vi "Dist Build App from LLB (proxy).vi"(4 "include run-time DLL":bool, 5 "active x server":string, 6 "mac mem size (k)":u32, 7 "lvrt res flags":i32, 8 "error in":errorcluster, 11 "paths":T1) -> (0 "error out":errorcluster)   [LabVIEW 2009]
doc: "\"Call By Reference\" proxy for .\\project\\prodisttol.llb\\Dist Build App from LLB.vi"
panel:
  in  "LV6.1 VI Refnum (for type)":refnum<vi>
  in  "LV7 VI Refnum (for type)":refnum<vi>
  in  "VI Refnum (for type)":refnum<vi>
  # "Dist Build App from LLB (proxy).vi\n\n\"Call By Reference\" proxy for .\\project\\prodisttol.llb\\Dist Build App from LLB.vi\n\nPlease visit http://www.OpenG.org to learn about the\nOpen Source LabVIEW software movement.\n\nNOTICE -- YOU MUST LEAVE THIS NOTICE IN PLACE.  PER THE TERMS OF THE LICENSE BELOW, YOU MAY SUBLICENSE THIS SOFTWARE \nIN ANY WAY THAT DOES NOT CONFLICT WITH THIS LICENSE.\n\n### BSD License (http://www.opensource.org/licenses/bsd-license.php) Begin ###\n \nCopyright (c) 2002, Jim Kring <jim@jimkring.com>\n\nAll rights reserved.\n\nRedistribution and use in source and binary forms, with or without modification, are permitted provided that the following conditions are met:\n\n    * Redistributions of source code must retain the above copyright notice, this list of conditions and the following disclaimer.\n    * Redistributions in binary form must reproduce the above copyright notice, this list of conditions and the following disclaimer in the \n       documentation and/or other materials provided with the distribution.\n    * Neither the name of SciWare, James Kring, Inc., nor the names of its contributors may be used to endorse or promote products derived \n       from this software without specific prior written permission.\n\nTHIS SOFTWARE IS PROVIDED BY THE COPYRIGHT HOLDERS AND CONTRIBUTORS \"AS IS\" AND ANY EXPRESS OR IMPLIED WARRANTIES, \nINCLUDING, BUT NOT LIMITED TO, THE IMPLIED WARRANTIES OF MERCHANTABILITY AND FITNESS FOR A PARTICULAR PURPOSE ARE \nDISCLAIMED. IN NO EVENT SHALL THE COPYRIGHT OWNER OR CONTRIBUTORS BE LIABLE FOR ANY DIRECT, INDIRECT, INCIDENTAL,\n SPECIAL, EXEMPLARY, OR CONSEQUENTIAL DAMAGES (INCLUDING, BUT NOT LIMITED TO, PROCUREMENT OF SUBSTITUTE GOODS OR \nSERVICES; LOSS OF USE, DATA, OR PROFITS; OR BUSINESS INTERRUPTION) HOWEVER CAUSED AND ON ANY THEORY OF LIABILITY, \nWHETHER IN CONTRACT, STRICT LIABILITY, OR TORT (INCLUDING NEGLIGENCE OR OTHERWISE) ARISING IN ANY WAY OUT OF THE USE \nOF THIS SOFTWARE, EVEN IF ADVISED OF THE POSSIBILITY OF SUCH DAMAGE.\n\n### BSD License End ###"
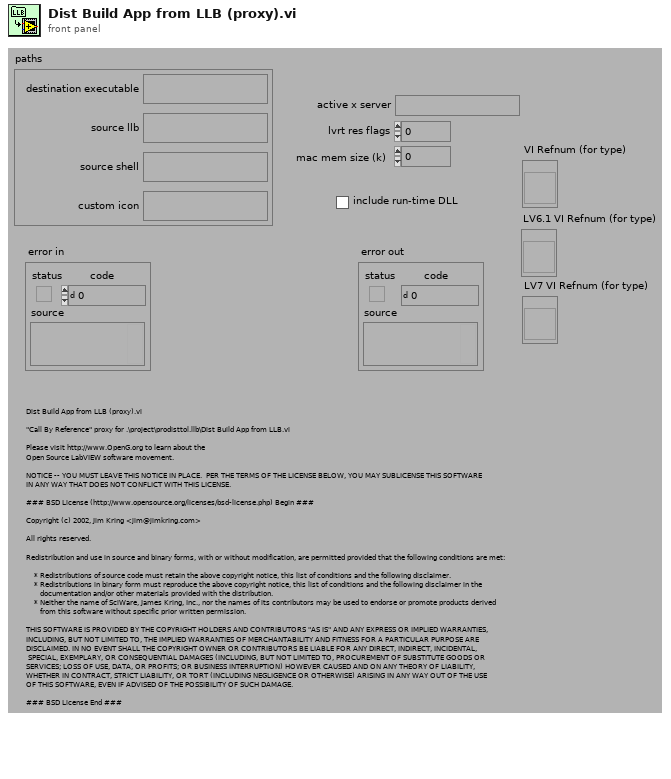
[diagram p1: front panel]
types:
  T1 = cluster{"destination executable":path, "source llb":path, "source shell":path, "custom icon":path}
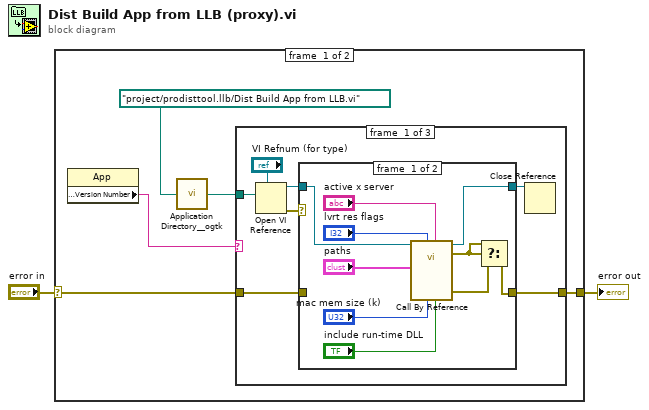
[diagram p0: block diagram]
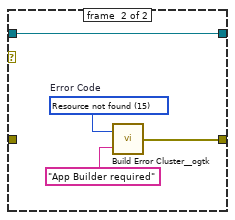
[diagram p2: hidden frame]
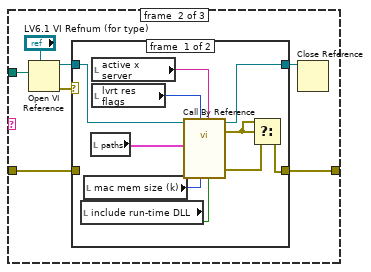
[diagram p3: hidden frame]
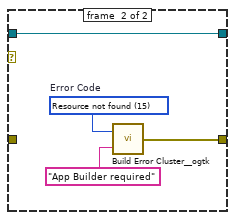
[diagram p4: hidden frame]
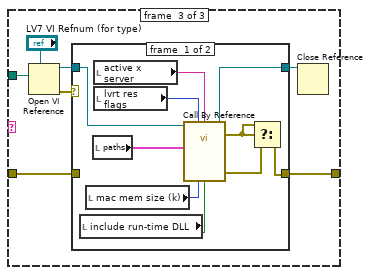
[diagram p5: hidden frame]
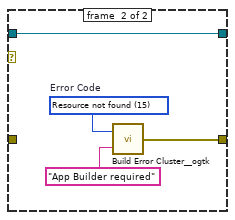
[diagram p6: hidden frame]
diagram:
  n1 = case shown="No Error" "error in" {
    selector: "error in" -> [w7 w71]
    tunnel: [w6 w71] -> w1
    frame #0 {
      n2 = property class="App"() -> ("Application:Version Number"=w5:string)  [unwired: 2 in, 2 out]
      n3 = call <userlib>:"Application Directory__ogtk.vi"("Relative path (.)"=path "project/prodisttool.llb/Dist Build App from LLB.vi") -> ("Application Directory (+ Relative)"=w4:path)
      n4 = case shown="\"6.0\", \"6.0.1\", \"6.0.2\"" w5 {
        tunnel: w4 -> [w14 w35 w56]
        tunnel: w7 -> [w12 w33 w54]
        tunnel: [w11 w32 w53] -> w6
        frame #0 {
          n5 = Open VI Reference(type specifier VI Refnum (for type only)="VI Refnum (for type)", vi path=w14) -> (vi reference=w10:refnum<vi>, error out=w13:errorcluster)  [unwired: 4 in]
          n6 = case shown="No Error" w13 {
            tunnel: w12 -> [_ _]
            tunnel: [w15 w27] -> w11
            tunnel: w10 -> [w24 w26]
            tunnel: [w18 w26] -> w8
            frame #0 {
              n7 = call-by-ref "?"(reference=w24, "include run-time DLL"="include run-time DLL", "active x server"="active x server", "mac mem size (k)"="mac mem size (k)", "lvrt res flags"="lvrt res flags", "paths"="paths") -> (reference out=w18:refnum<vi>, error out=w17:errorcluster, "error out"=w16:errorcluster)  [unwired: 7 in]
              n8 = Select(t=w17, s=w17, f=w16) -> (s? t:f=w15:errorcluster)
            }
            frame #1 {
              w25 = u16 15 items=["No error", "Argument error", "Memory is full", "Out of zone", "End of file", "File already open", "Generic file I/O error", "File not found", "File permission error", "Disk is full", "Duplicate path", "Too many files open", "System feature not enabled", "Resource file not found", "Cannot add resource", "Resource not found", "Image not found", "Image memory error", "Pen does not exist", "Config type invalid", "Config token not found", "Config parse error", "Config memory error", "Bad external code format", "Bad external code offset", "External code not present", "Null window", "Destroy window error", "Null menu", "Print aborted", "Bad print record", "Print driver error", "Windows error during printing", "Memory error during printing", "Print dialog error", "Generic print error", "Invalid device refnum", "Device not found", "Device parameter error", "Device unit error", "Cannot open device", "Device call aborted", "Generic error", "Cancelled by user", "Object ID too low", "Object ID too high", "Object not in heap", "Unknown heap", "Unknown object (invalid DefProc)", "Unknown object (DefProc not in table)", "Message out of range", "Invalid (null) method", "Unknown message", "Manager call not supported", "Bad address", "Network operation in progress", "Network operation timed out", "Connection is busy", "Network attribute not supported", "Network error", "Address in use", "System out of memory", "Connection aborted", "Connection refused", "Not connected", "Already connected", "Connection closed", "Initialization error (interapplication manager)", "Bad occurrence", "Wait on unbound occurrence handler", "Occurrence queue overflow", "Datalog type conflict", "Unused", "Unrecognized type (interapplication manager)", "Memory corrupt", "Failed to make temporary DLL", "Old CIN version", "Drag socket not found", "Failed to load drop-object", "Failed to register OLE object", "Failed to release OLE object", "Format specifier type mismatch", "Unknown format specifier", "Too few format specifiers", "Too many format specifiers", "Scan failed", "Newer CIN version", "OLE Convert", "Runtime menu error", "Password tampered", "Unknown error code"]  # Error Code
              n9 = call <userlib>:"Build Error Cluster__ogtk.vi"("String to Prepend to source (\"\")"="App Builder required" ("String to Prepend to source (\"\")"), "code"=w25) -> ("error out"=w27:errorcluster)
            }
          }
          n10 = Close Reference(reference=w8) -> ()  [unwired: 1 in, 1 out]
        }
        frame #1 {
          n11 = Open VI Reference(type specifier VI Refnum (for type only)="LV6.1 VI Refnum (for type)", vi path=w35) -> (vi reference=w31:refnum<vi>, error out=w34:errorcluster)  [unwired: 4 in]
          n12 = case shown="No Error" w34 {
            tunnel: w33 -> [_ _]
            tunnel: [w41 w48] -> w32
            tunnel: w31 -> [w45 w47]
            tunnel: [w44 w47] -> w30
            frame #0 {
              n13 = local read "include run-time DLL"() -> (w38:bool)
              n14 = local read "mac mem size (k)"() -> (w37:u32)
              n15 = local read "paths"() -> (w36:T1)
              n16 = local read "active x server"() -> (w40:string)
              n17 = local read "lvrt res flags"() -> (w39:i32)
              n18 = call-by-ref "?"(reference=w45, "include run-time DLL"=w38, "active x server"=w40, "mac mem size (k)"=w37, "lvrt res flags"=w39, "paths"=w36) -> (reference out=w44:refnum<vi>, error out=w43:errorcluster, "error out"=w42:errorcluster)  [unwired: 7 in]
              n19 = Select(t=w43, s=w43, f=w42) -> (s? t:f=w41:errorcluster)
            }
            frame #1 {
              w46 = u16 15 items=["No error", "Argument error", "Memory is full", "Out of zone", "End of file", "File already open", "Generic file I/O error", "File not found", "File permission error", "Disk is full", "Duplicate path", "Too many files open", "System feature not enabled", "Resource file not found", "Cannot add resource", "Resource not found", "Image not found", "Image memory error", "Pen does not exist", "Config type invalid", "Config token not found", "Config parse error", "Config memory error", "Bad external code format", "Bad external code offset", "External code not present", "Null window", "Destroy window error", "Null menu", "Print aborted", "Bad print record", "Print driver error", "Windows error during printing", "Memory error during printing", "Print dialog error", "Generic print error", "Invalid device refnum", "Device not found", "Device parameter error", "Device unit error", "Cannot open device", "Device call aborted", "Generic error", "Cancelled by user", "Object ID too low", "Object ID too high", "Object not in heap", "Unknown heap", "Unknown object (invalid DefProc)", "Unknown object (DefProc not in table)", "Message out of range", "Invalid (null) method", "Unknown message", "Manager call not supported", "Bad address", "Network operation in progress", "Network operation timed out", "Connection is busy", "Network attribute not supported", "Network error", "Address in use", "System out of memory", "Connection aborted", "Connection refused", "Not connected", "Already connected", "Connection closed", "Initialization error (interapplication manager)", "Bad occurrence", "Wait on unbound occurrence handler", "Occurrence queue overflow", "Datalog type conflict", "Unused", "Unrecognized type (interapplication manager)", "Memory corrupt", "Failed to make temporary DLL", "Old CIN version", "Drag socket not found", "Failed to load drop-object", "Failed to register OLE object", "Failed to release OLE object", "Format specifier type mismatch", "Unknown format specifier", "Too few format specifiers", "Too many format specifiers", "Scan failed", "Newer CIN version", "OLE Convert", "Runtime menu error", "Password tampered", "Unknown error code"]  # Error Code
              n20 = call <userlib>:"Build Error Cluster__ogtk.vi"("String to Prepend to source (\"\")"="App Builder required" ("String to Prepend to source (\"\")"), "code"=w46) -> ("error out"=w48:errorcluster)
            }
          }
          n21 = Close Reference(reference=w30) -> ()  [unwired: 1 in, 1 out]
        }
        frame #2 {
          n22 = Open VI Reference(type specifier VI Refnum (for type only)="LV7 VI Refnum (for type)", vi path=w56) -> (vi reference=w52:refnum<vi>, error out=w55:errorcluster)  [unwired: 4 in]
          n23 = case shown="Error" w55 {
            tunnel: w54 -> [_ _]
            tunnel: [w64 w69] -> w53
            tunnel: w52 -> [w63 w68]
            tunnel: [w57 w68] -> w51
            frame #0 {
              n24 = local read "include run-time DLL"() -> (w59:bool)
              n25 = local read "mac mem size (k)"() -> (w58:u32)
              n26 = local read "paths"() -> (w60:T1)
              n27 = local read "active x server"() -> (w62:string)
              n28 = local read "lvrt res flags"() -> (w61:i32)
              n29 = call-by-ref "?"(reference=w63, "paths"=w60, "lvrt res flags"=w61, "active x server"=w62, "mac mem size (k)"=w58, "include run-time DLL"=w59) -> (reference out=w57:refnum<vi>, error out=w66:errorcluster, "error out"=w65:errorcluster)  [unwired: 10 in, 1 out]
              n30 = Select(t=w66, s=w66, f=w65) -> (s? t:f=w64:errorcluster)
            }
            frame #1 {
              w67 = u16 15 items=["No error", "Argument error", "Memory is full", "Out of zone", "End of file", "File already open", "Generic file I/O error", "File not found", "File permission error", "Disk is full", "Duplicate path", "Too many files open", "System feature not enabled", "Resource file not found", "Cannot add resource", "Resource not found", "Image not found", "Image memory error", "Pen does not exist", "Config type invalid", "Config token not found", "Config parse error", "Config memory error", "Bad external code format", "Bad external code offset", "External code not present", "Null window", "Destroy window error", "Null menu", "Print aborted", "Bad print record", "Print driver error", "Windows error during printing", "Memory error during printing", "Print dialog error", "Generic print error", "Invalid device refnum", "Device not found", "Device parameter error", "Device unit error", "Cannot open device", "Device call aborted", "Generic error", "Cancelled by user", "Object ID too low", "Object ID too high", "Object not in heap", "Unknown heap", "Unknown object (invalid DefProc)", "Unknown object (DefProc not in table)", "Message out of range", "Invalid (null) method", "Unknown message", "Manager call not supported", "Bad address", "Network operation in progress", "Network operation timed out", "Connection is busy", "Network attribute not supported", "Network error", "Address in use", "System out of memory", "Connection aborted", "Connection refused", "Not connected", "Already connected", "Connection closed", "Initialization error (interapplication manager)", "Bad occurrence", "Wait on unbound occurrence handler", "Occurrence queue overflow", "Datalog type conflict", "Unused", "Unrecognized type (interapplication manager)", "Memory corrupt", "Failed to make temporary DLL", "Old CIN version", "Drag socket not found", "Failed to load drop-object", "Failed to register OLE object", "Failed to release OLE object", "Format specifier type mismatch", "Unknown format specifier", "Too few format specifiers", "Too many format specifiers", "Scan failed", "Newer CIN version", "OLE Convert", "Runtime menu error", "Password tampered", "Unknown error code"]  # Error Code
              n31 = call <userlib>:"Build Error Cluster__ogtk.vi"("String to Prepend to source (\"\")"="App Builder required" ("String to Prepend to source (\"\")"), "code"=w67) -> ("error out"=w69:errorcluster)
            }
          }
          n32 = Close Reference(reference=w51) -> ()  [unwired: 1 in, 1 out]
        }
      }
    }
    frame #1 {
    }
  }
  "error out" <- w1
